vi "PS4 Controller - Polling Read.vi"() -> ()   [LabVIEW 2020, in "LMH-PS4.lvlib"]
doc: "This example demonstrates how to read from a Play Station 4 controller using polling."
uses:
  LMH-PS4.lvlib
  Private/Type Defs/Indicators/Controller.ctl
  Private/Type Defs/Indicators/Square.ctl
  Private/Type Defs/Indicators/X.ctl
  Private/Type Defs/Indicators/Circle.ctl
  Private/Type Defs/Indicators/Triangle.ctl
  Private/Type Defs/Indicators/L1.ctl
  Private/Type Defs/Indicators/R1.ctl
  Private/Type Defs/Indicators/Share.ctl
  Private/Type Defs/Indicators/Options.ctl
  Private/Type Defs/Indicators/PS.ctl
  Private/Type Defs/Indicators/Pad_Button.ctl
  Private/Type Defs/Indicators/Dpad.ctl
  Private/Type Defs/Indicators/Slider.ctl
  Public/Open First Controller.vi
  <vilib>/ReMiSYS Technology/RemoteToolkit/Sender/Sender.lvclass
panel:
  in  "IP Address":string="10.12.34.2"
  out "PS4 Controller":T1={"Square Button"=FALSE, "X Button"=FALSE, "Circle Button"=FALSE, "Triangle Button"=FALSE, "L1"=FALSE, "R1"=FALSE, "Share Button"=FALSE, "Options Button"=FALSE, "PS Button"=FALSE, "Pad Button"=FALSE, "D-Pad"=5, "L2"=0, "R2"=0, "Thumbstick_Left"={[], []}, "Thumbstick_Right"={[], []}} {"R2" scale=-32768.0..32767.0; "L2" scale=-32768.0..32767.0}
  in  "Stop Button":bool
  # "Controller Data"
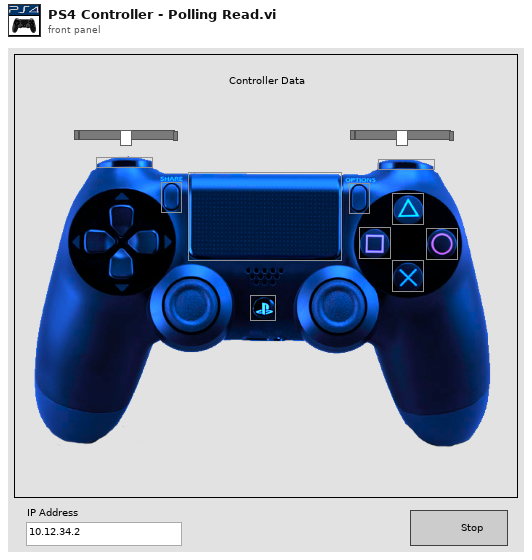
[diagram p1: front panel]
types:
  T1 = typedef "LMH-PS4.lvlib/Controller.ctl" = cluster{"Square Button":T2, "X Button":T3, "Circle Button":T4, "Triangle Button":T5, "L1":T6, "R1":T7, "Share Button":T8, "Options Button":T9, "PS Button":T10, "Pad Button":T11, "D-Pad":T12, "L2":T13, "R2":T13, "Thumbstick_Left":cluster{i32[], i32[]}, "Thumbstick_Right":cluster{i32[], i32[]}}
  T2 = typedef "LMH-PS4.lvlib/Square.ctl" = bool
  T3 = typedef "LMH-PS4.lvlib/X.ctl" = bool
  T4 = typedef "LMH-PS4.lvlib/Circle.ctl" = bool
  T5 = typedef "LMH-PS4.lvlib/Triangle.ctl" = bool
  T6 = typedef "LMH-PS4.lvlib/L1.ctl" = bool
  T7 = typedef "LMH-PS4.lvlib/R1.ctl" = bool
  T8 = typedef "LMH-PS4.lvlib/Share.ctl" = bool
  T9 = typedef "LMH-PS4.lvlib/Options.ctl" = bool
  T10 = typedef "LMH-PS4.lvlib/PS.ctl" = bool
  T11 = typedef "LMH-PS4.lvlib/Pad_Button.ctl" = bool
  T12 = typedef "LMH-PS4.lvlib/Dpad.ctl" = u16
  T13 = typedef "LMH-PS4.lvlib/Slider.ctl" = i32
  T14 = typedef "LMH-PS4.lvlib/PS4 Controller Ref.ctl" = cluster{"Controller Ref":refnum<k1>, "PS4 Events Ref":refnum<event-registration>, "Worker Ref":refnum<vi>}
  T15 = typedef "LMH-PS4.lvlib/Axis.ctl" = cluster{"Left Thumbstick":cluster{"X Axis":i32, "Y Axis":i32}, "Right Thumbstick":cluster{"X Axis":i32, "Y Axis":i32}, "L2":i32, "R2":i32, "D-Pad":T16}
  T16 = typedef "LMH-PS4.lvlib/DPad Enum.ctl" = enum16{"Idle", "Up", "Up / Right", "Right", "Down / Right", "Down", "Down / Left", "Left", "Up / Left"}
  T17 = typedef "LMH-PS4.lvlib/Buttons.ctl" = cluster{"Square":bool, "X":bool, "Circle":bool, "Triangle":bool, "L1":bool, "R1":bool, "L2":bool, "R2":bool, "Share":bool, "Options":bool, "Left Thumbstick":bool, "Right Thumbstick":bool, "Playstation Button":bool, "Pad":bool}
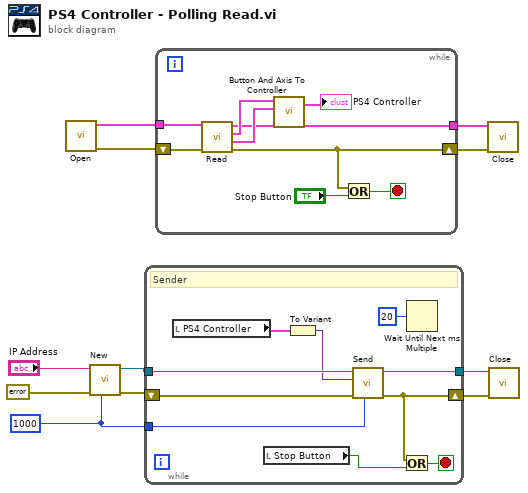
[diagram p0: block diagram]
diagram:
  w5 = 1000 ("Timeout ms (25000)")
  n1 = call-poly "Open.vi"() -> ("Error Out"=w9:errorcluster, "PS4 Controller Ref"=w8:T14)  [unwired: 9 in, 1 out]
  n2 = call <vilib>:"New.vi"("Timeout ms (25000)"=w5, "Error In"=errorcluster {"status"=FALSE, "code"=0, "source"=""}, "IP Address"="IP Address") -> ("Error Out"=w6:errorcluster, "Sender Ref."=w3:refnum<class "Sender.lvclass">)  [unwired: 7 in]
  n3 = while {
    shift-right: [w17] -> w2
    shift-left: w6 -> [w19]
    tunnel: w3 -> [w20]
    tunnel: w5 -> [w15]
    tunnel: [w18] -> w1
    stop <- w21 stop-if-true
    # "Sender"
    n4 = local read "PS4 Controller"() -> (w13:T1)
    n5 = local read "Stop Button"() -> (w12:bool)
    n6 = To Variant(anything=w13) -> (Variant=w16:variant)
    n7 = call <vilib>:"Send.vi"("Timeout ms (1000)"=w15, "Error In"=w19, "Value"=w16, "Sender Ref."=w20) -> ("Error Out"=w17:errorcluster, "Sender Ref."=w18:refnum<class "Sender.lvclass">)  [unwired: 6 in]
    n8 = Or(x=w17, y=w12) -> (x .or. y?=w21:bool)
    n9 = Wait Until Next ms Multiple(millisecond multiple=u32 20) -> ()  [unwired: 1 out]
  }
  n10 = while {
    shift-right: [w26] -> w11
    shift-left: w9 -> [w23]
    tunnel: [w25] -> w10
    tunnel: w8 -> [w24]
    stop <- w28 stop-if-true
    n11 = call "Read.vi"("Error In"=w23, "PS4 Controller Ref"=w24) -> ("Error Out"=w26:errorcluster, "All Axis"=w30:T15, "Buttons"=w29:T17, "PS4 Controller Ref"=w25:T14)  [unwired: 6 in]
    n12 = call "Button And Axis To Controller.vi"("All Axis"=w30, "Buttons"=w29) -> ("PS4 Controller"=→"PS4 Controller":T1)  [unwired: 5 in]
    n13 = Or(x=w26, y="Stop Button") -> (x .or. y?=w28:bool)
  }
  n14 = call <vilib>:"Close.vi"("Error In"=w11, "PS4 Controller Ref"=w10) -> ()  [unwired: 9 in, 1 out]
  n15 = call <vilib>:"Close.vi"("Error In"=w2, "Receiver Ref."=w1) -> ()  [unwired: 9 in, 1 out]
